vi "My_Controls_Example_With_MathScript.vi"() -> ()   [LabVIEW 2022 SP3]
panel:
  in  "stop":bool
  out "Step Response Graph":cdb[](graph)
  in  "Natural Frequency":dbl(slide) scale=0.0..5.0
  in  "Damping Ratio":dbl(slide) scale=0.0..1.0
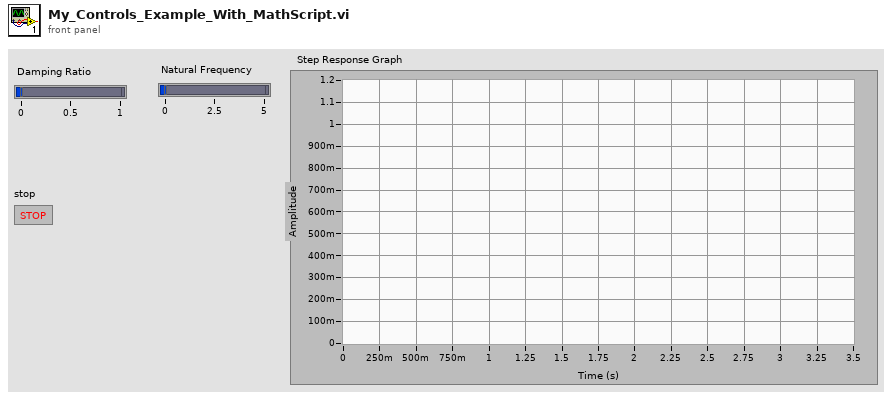
[diagram p1: front panel]
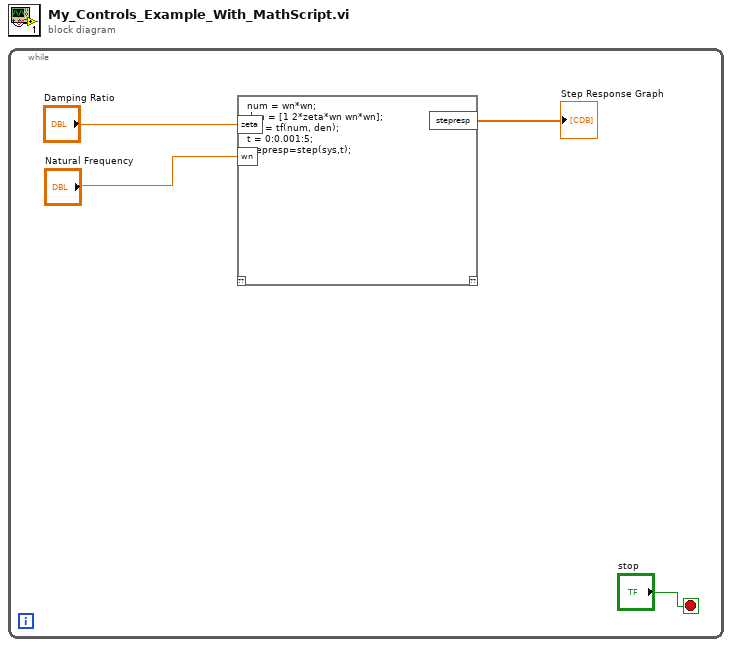
[diagram p0: block diagram]
diagram:
  n1 = while {
    stop <- "stop" stop-if-true
    n2 = script code="num = wn*wn;\nden = [1 2*zeta*wn wn*wn];\nsys = tf(num, den);\nt = 0:0.001:5;\nstepresp=step(sys,t);" ("Script Node")("zeta"="Damping Ratio", "wn"="Natural Frequency") -> ("stepresp"=→"Step Response Graph":cdb[])  [unwired: 1 in, 1 out]
  }
